vi "Create Paramaterized Executive.vi"(8 "error in (no error)":errorcluster, 10 "Create Paramaterized Executive":T1, 11 "Test Executive Builder in":refnum<class "Test Executive Builder.lvclass">) -> (0 "error out":errorcluster, 3 "Test Executive Builder out":refnum<class "Test Executive Builder.lvclass">)   [LabVIEW 2019, in "Test Executive Builder.lvclass"]
uses:
  <vilib>/gpm_packages/@cs/Test-executive-builder/Example/Application/Test Executive Builder/Test Executive Builder/Test Executive Builder.lvclass
  C:/Program Files/National Instruments/LabVIEW 2019/vi.lib/gpm_packages/@cs/Test-executive-builder/Source/Test Executive Builder Model/Test Executive Builder Model/Test Executive Builder Model.lvclass
  C:/Program Files/National Instruments/LabVIEW 2019/vi.lib/gpm_packages/@cs/mva-core/Source/IModel/IModel/IModel.lvclass
  <vilib>/gpm_packages/@cs/Test-executive-builder/Source/Application Dependencies/Create Paramaterized Executive.ctl
  <vilib>/gpm_packages/@cs/Test-executive-builder/Source/Test Executive Builder Model/Test Executive Builder Model/Test Executive Builder Model.lvclass/Test Executive Builder Model.ctl
  <vilib>/gpm_packages/@cs/Test-executive-builder/Example/Application/Test Executive Builder/Test Executive Builder/Test Executive Builder.lvclass/Test Executive Builder.ctl
  <vilib>/gpm_packages/@cs/mva-core/Source/IObserver/IObserver/IObserver.lvclass/IObserver.ctl
  <vilib>/gpm_packages/@cs/mva-core/Source/IModel/IModel/IModel.lvclass/IModel.ctl
  <vilib>/gpm_packages/@cs/mva-core/Source/IMediator/PublishRequest/PublishRequest.lvclass/PublishRequest.ctl
  <vilib>/gpm_packages/@cs/mva-core/Source/IMediator/IMediator Messages/Publish Msg/Publish Msg.lvclass/Publish Msg.ctl
  <vilib>/gpm_packages/@cs/actor-framework-messages/Source/RoundTripMessage/RoundTripMessage.lvclass/RoundTripMessage.ctl
  <vilib>/ActorFramework/Message Enqueuer/Message Enqueuer.lvclass/Message Enqueuer.ctl
  37f1e1d7-7973-4b43-9f61-0c22a5b43bb0.vi
  <vilib>/gpm_packages/@cs/mva-core/Source/IMediator/IMediator Messages/Publish Msg/Send Pre-Addressed Publish.vi
  <vilib>/gpm_packages/@cs/mva-core/Source/IObserver/IObserver/Read Unique ID.vi
  <vilib>/gpm_packages/@cs/mva-core/Source/IMediator/PublishRequest/Pack Publish Request.vi
  <vilib>/gpm_packages/@cs/actor-framework-messages/Source/RoundTripMessage/Return Round-Trip Message.vi
  <vilib>/ActorFramework/Message Enqueuer/Enqueue.vi
  <vilib>/gpm_packages/@cs/mva-core/Source/IModel/IModel/IModel.lvclass
  C:/Program Files/National Instruments/LabVIEW 2019/vi.lib/gpm_packages/@cs/mva-core/Source/IObserver/IObserver/IObserver.lvclass
  <vilib>/gpm_packages/@cs/mva-core/Source/IMediator/IMediator Messages/Publish Msg/Publish Msg.lvclass
  C:/Program Files/National Instruments/LabVIEW 2019/vi.lib/gpm_packages/@cs/actor-framework-messages/Source/RoundTripMessage/RoundTripMessage.lvclass
  <vilib>/gpm_packages/@cs/actor-framework-messages/Source/RoundTripMessage/RoundTripMessage.lvclass
  C:/Program Files/National Instruments/LabVIEW 2019/vi.lib/ActorFramework/Message/Message.lvclass
  <vilib>/Utility/error.llb/Error Cluster From Error Code.vi
  <vilib>/ActorFramework/Message Priority Queue/Priority Enqueue.vi
  <vilib>/gpm_packages/@cs/test-executive/Source/Test Executive/ITestExecutive/ITest Executive.lvclass
  <vilib>/gpm_packages/@cs/mva-core/Source/IMediator/PublishRequest/PublishRequest.lvclass
  <vilib>/gpm_packages/@cs/test-executive/Source/Test Executive/TestExecutive Ref/TestExecutive Ref.lvclass
  <vilib>/gpm_packages/@cs/Test-executive-builder/Source/Test Executive Builder Model/Test Executive Builder Model/Test Executive Builder Model.lvclass
  <vilib>/gpm_packages/@cs/Test-executive-builder/Source/Test Executive Builder Dialogs/ITest Executive Builder Dialog/ITest Executive Builder Dialog.lvclass
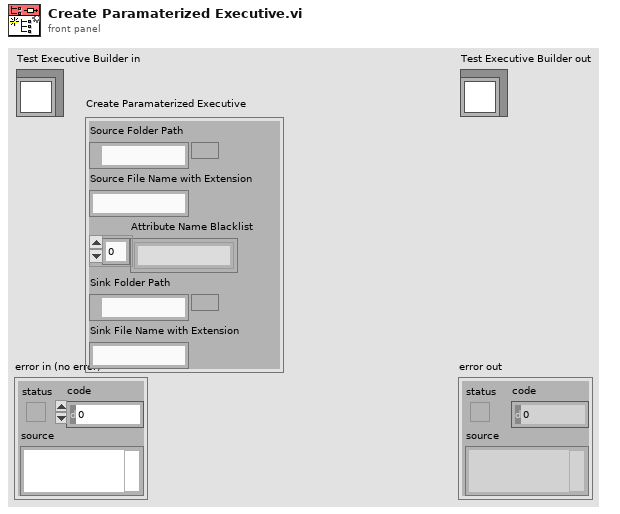
[diagram p1: front panel]
types:
  T1 = typedef "Create Paramaterized Executive.ctl" = cluster{"Source Folder Path":path, "Source File Name with Extension":string, "Attribute Name Blacklist":string[], "Sink Folder Path":path, "Sink File Name with Extension":string}
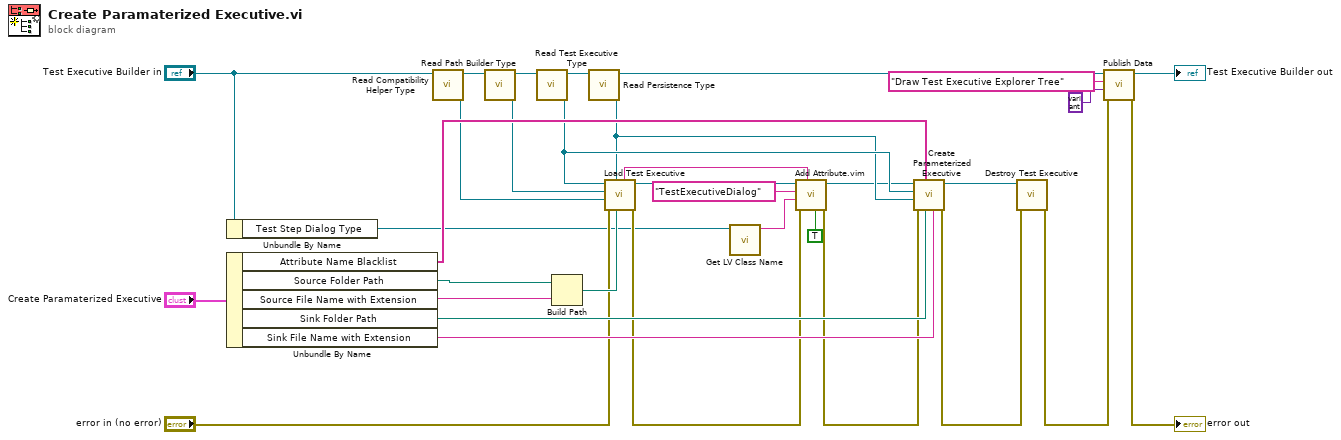
[diagram p0: block diagram]
diagram:
  n1 = Unbundle By Name("Test Executive Builder in") -> ("Test Step Dialog Type"=w1:refnum<class "ITest Executive Builder Dialog.lvclass">)
  n2 = Unbundle By Name("Create Paramaterized Executive") -> ("Attribute Name Blacklist"=w30:string[], "Source Folder Path"=w32:path, "Source File Name with Extension"=w31:string, "Sink Folder Path"=w27:path, "Sink File Name with Extension"=w26:string)
  n3 = call <vilib>:"Read Compatibility Helper Type.vi"("Test Executive Builder Model in"="Test Executive Builder in") -> ("Compatibility Helper"=w20:refnum<class "ICompatibility Helper.lvclass">, "Test Executive Builder Model out"=w24:refnum<class "Test Executive Builder.lvclass">)  [unwired: 9 in]
  n4 = call <vilib>:"Read Path Builder Type.vi"("Test Executive Builder Model in"=w24) -> ("Path Builder"=w19:refnum<class "IPath Builder.lvclass">, "Test Executive Builder Model out"=w23:refnum<class "Test Executive Builder.lvclass">)  [unwired: 9 in]
  n5 = call <vilib>:"Read Test Executive Type.vi"("Test Executive Builder Model in"=w23) -> ("Test Executive"=w18:refnum<class "ITest Executive.lvclass">, "Test Executive Builder Model out"=w22:refnum<class "Test Executive Builder.lvclass">)  [unwired: 9 in]
  n6 = Build Path(base path=w32, name or relative path=w31) -> (appended path=w33:path)
  n7 = call <vilib>:"Read Persistence Type.vi"("Test Executive Builder Model in"=w22) -> ("Persist"=w17:refnum<class "IPersist.lvclass">, "Test Executive Builder Model out"=w6:refnum<class "Test Executive Builder.lvclass">)  [unwired: 9 in]
  n8 = call <vilib>:"Load Test Executive.vi"("Folder"=w33, "Persistence in"=w17, "error in (no error)"="error in (no error)", "Compatibility Helper"=w20, "Path Builder"=w19, "Test Executive"=w18) -> ("error out"=w13:errorcluster, "Test Executive Ref out"=w16:refnum<data-value>, "Root ID"=w14:string)  [unwired: 3 in]
  n9 = call <vilib>:"Get LV Class Name.vi"("object"=w1) -> ("class name"=w9:string)  [unwired: 9 in, 1 out]
  n10 = call "Add Attribute.vim"("Private?"=TRUE, "ID"=w14, "error in (no error)"=w13, "Attribute"=w9, "Attribute Name"="TestExecutiveDialog", "Test Executive Ref"=w16) -> ("error out"=w12:errorcluster, "Test Executive Ref out"=w15:refnum<data-value>)  [unwired: 2 in, 2 out]
  n11 = call <vilib>:"Create Parameterized Executive.vi"("File Name"=w26, "Folder"=w27, "Attribute Name Blacklist"=w30, "error in (no error)"=w12, "Persistence in"=w17, "Test Executive"=w18, "Test Executive Ref"=w15) -> ("error out"=w28:errorcluster, "Test Executive Ref out"=w29:refnum<data-value>)  [unwired: 3 in]
  n12 = call <vilib>:"Destroy Test Executive.vi"("error in (no error)"=w28, "Test Executive Ref"=w29) -> ("error out"=w4:errorcluster)  [unwired: 9 in]
  n13 = call <vilib>:"Publish Data.vi"("error in (no error)"=w4, "Data to Publish"=variant ("Data Type"), "Datum Name"="Draw Test Executive Explorer Tree", "IModel in"=w6) -> ("error out"=→"error out":errorcluster, "IModel out"=→"Test Executive Builder out":refnum<class "Test Executive Builder.lvclass">)  [unwired: 6 in]
